vi "NewBusNumber.vi"(8 "ErrorArray In":errorcluster[](array[cluster])) -> (0 "ErrorArray Out":errorcluster[](array[cluster]), 1 "BusNumber":u8)   [LabVIEW 2017, in "Framework.lvlib"]
uses:
  Framework.lvlib
  <vilib>/Utility/error.llb/Error Cluster From Error Code.vi
  <vilib>/ErrorRing/Error Ring.xnode
  <userlib>/NIST/NISTErrorLib/NISTErrorLib.lvlib
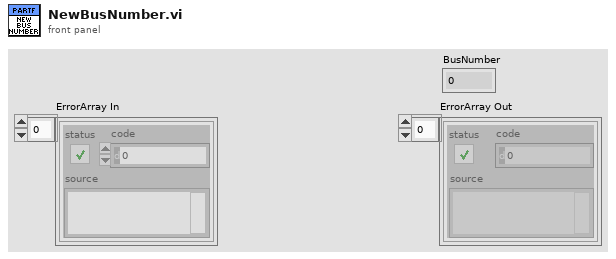
[diagram p1: front panel]
types:
  T1 = typedef "Framework.lvlib/clFrontPanelControlRefs.ctl" = cluster{"TestFilePathRef":refnum<vi>, "BusNumberRef":refnum<vi>, "NumberOfBusesRef":refnum<vi>, "EvtTypeRef":refnum<vi>, "EvtParamsRef":refnum<vi>, "EvtConfigRef":refnum<vi>, "StartTimeRef":refnum<vi>, "EndTimeRef":refnum<vi>, "PmuImpairTypeRef":refnum<vi>, "PmuImpairParamsRef":refnum<vi>, "NetImpairParamsRef":refnum<vi>, "FlagImpairTypeRef":refnum<vi>, "FlagImpairParamsRef":refnum<vi>, "NetImpairTypeRef":refnum<vi>, "OutputFileType":refnum<vi>, "PmuImpairConfigRef":refnum<vi>, "AppTypeRef":refnum<vi>, "ScriptPathRef":refnum<vi>, "ShowPanels?":refnum<vi>}
  T2 = typedef "LVStringsAndValuesArrayTypeDef_U8.ctl" = cluster{"String":string, "Value":u8}[]
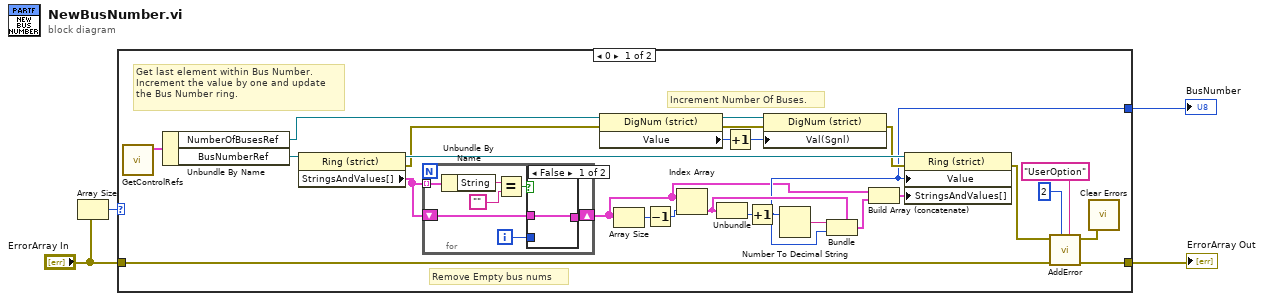
[diagram p0: block diagram]
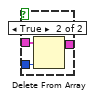
[diagram p2: hidden frame]
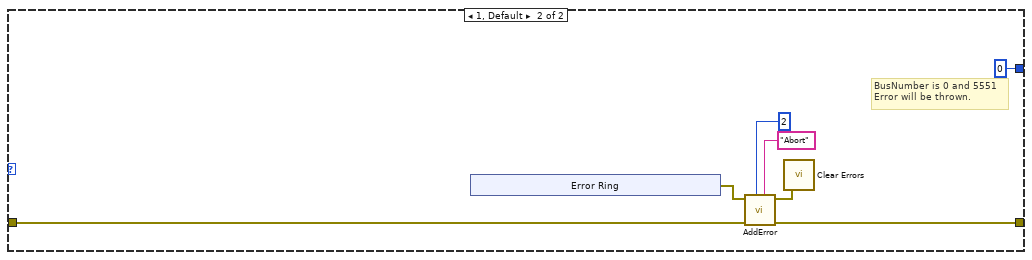
[diagram p3: hidden frame]
diagram:
  n1 = Array Size(array="ErrorArray In") -> (size(s)=w4:i32)
  n2 = case shown="0" w4 {
    tunnel: "ErrorArray In" -> [w30 w42]
    tunnel: [w29 w43] -> w1
    tunnel: [w8 u8 0] -> w2
    frame 0 {
      # "Remove Empty bus nums"
      # "Get last element within Bus Number.\nIncrement the value by one and update\nthe Bus Number ring."
      # "Increment Number Of Buses."
      n3 = call "GetControlRefs.vi"() -> ("clControlRefs Out"=w7:T1)  [unwired: 11 in]
      n4 = Unbundle By Name(w7) -> ("NumberOfBusesRef"=w21:refnum<vi>, "BusNumberRef"=w20:refnum<vi>)
      n5 = property class="Ring (strict)"(reference=w20) -> (reference out=w22:refnum<vi>, error out=w19:errorcluster, "StringsAndValues[]"=w6:T2)  [unwired: 1 in]
      n6 = for {
        tunnel: w6 -> [w37] mode=indexing
        shift-right: [w31] -> w5
        shift-left: w6 -> [w33]
        i -> [w32]
        n7 = Unbundle By Name(w37) -> ("String"=w36:string)
        n8 = Equal?(x=w36, y="") -> (x = y?=w34:bool)
        n9 = case shown="False" w34 {
          tunnel: w33 -> [w38 w41]
          tunnel: w32 -> [_ w40]
          tunnel: [w38 w39] -> w31
          frame False {
          }
          frame True {
            n10 = Delete From Array(array=w41, index=w40) -> (array with subset deleted=w39:T2)  [unwired: 1 in, 1 out]
          }
        }
      }
      n11 = property class="DigNum (strict)"(reference=w21, error in=w19) -> (reference out=w24:refnum<vi>, error out=w23:errorcluster, "Value"=w25:u8)
      n12 = Array Size(array=w5) -> (size(s)=w15:i32)
      n13 = Decrement(x=w15) -> (x-1=w14:i32)
      n14 = Index Array(array=w5, index=w14) -> (element=w12:cluster{"String":string, "Value":u8})
      n15 = Unbundle(w12) -> ("Value"=w13:u8)  [unwired: 1 out]
      n16 = Increment(x=w25) -> (x+1=w16:u8)
      n17 = Increment(x=w13) -> (x+1=w8:u8)
      n18 = property class="DigNum (strict)"(reference=w24, error in=w23, "Val(Sgnl)"=w16) -> (error out=w18:errorcluster)  [unwired: 1 out]
      n19 = Number To Decimal String(number=w8) -> (decimal integer string=w11:string)  [unwired: 1 in]
      n20 = Bundle(cluster=w12, "String"=w11, "Value"=w8) -> (w10:cluster{"String":string, "Value":u8})
      n21 = Build Array (concatenate)(w5, w10) -> (w9:T2)
      n22 = property class="Ring (strict)"(reference=w22, error in=w18, "Value"=w8, "StringsAndValues[]"=w9) -> (error out=w17:errorcluster)  [unwired: 1 out]
      n23 = call <userlib>:"AddError.vi"("Severity"="UserOption" ("String"), "Priority"=u8 2, "ErrorArray"=w30, "error in (no error)"=w17) -> ("ErrorArray"=w29:errorcluster[], "error out"=w28:errorcluster)  [unwired: 6 in]
      n24 = call <vilib>:"Clear Errors.vi"("error in (no error)"=w28) -> ()  [unwired: 5 in, 2 out]
    }
    frame 1, Default {
      # "BusNumber is 0 and 5551\nError will be thrown."
      n25 = xnode "Error Ring"() -> ("error out"=w44:errorcluster)
      n26 = call <userlib>:"AddError.vi"("Severity"="Abort" ("String"), "Priority"=u8 2, "ErrorArray"=w42, "error in (no error)"=w44) -> ("ErrorArray"=w43:errorcluster[], "error out"=w47:errorcluster)  [unwired: 6 in]
      n27 = call <vilib>:"Clear Errors.vi"("error in (no error)"=w47) -> ()  [unwired: 5 in, 2 out]
    }
  }
  "ErrorArray Out" <- w1
  "BusNumber" <- w2
